vi "Write Valve Parameters.vi"(7 "listen period":sgl=0.1, 8 "error in":errorcluster, 9 "Valve Range":i32=5391, 10 "Valve Offset":i32=13225, 11 "Brooks MFC in":refnum<class "Brooks MFC.lvclass">) -> (0 "error out":errorcluster, 1 "Valve Range":i32=5391, 2 "Valve Offset":i32=13225, 3 "Brooks MFC out":refnum<class "Brooks MFC.lvclass">)   [LabVIEW 2016, in "Brooks MFC.lvclass"]
uses:
  Brooks MFC.lvclass
  Brooks MFC.lvclass/Brooks MFC.ctl
  Instance           5 30Saved   Write Valve Parameters .vi
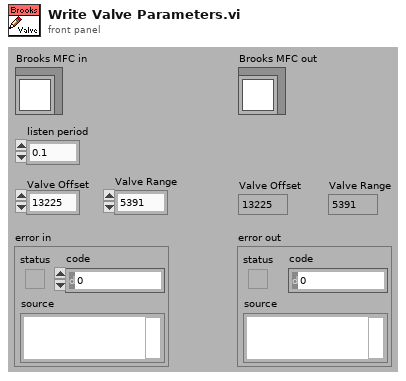
[diagram p1: front panel]
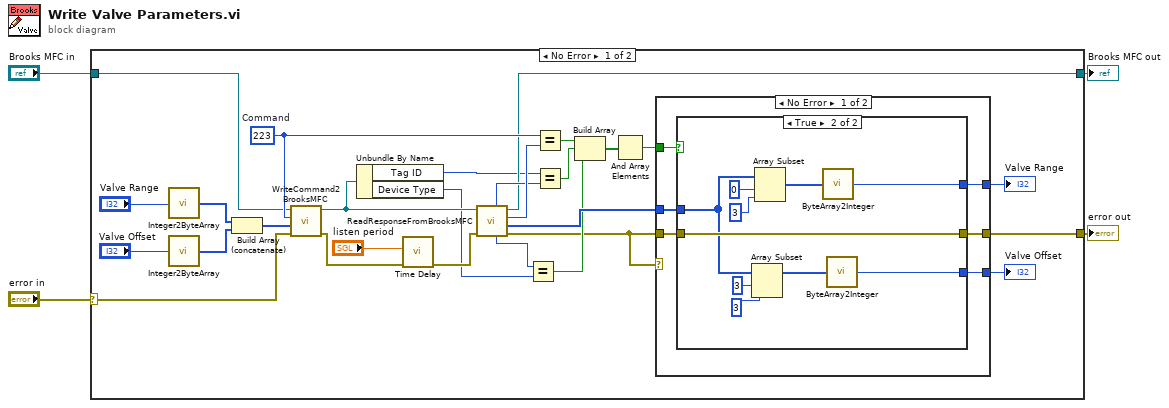
[diagram p0: block diagram]
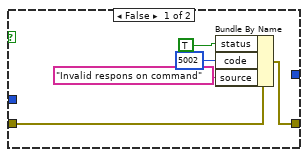
[diagram p2: hidden frame]
diagram:
  n1 = case shown="No Error" "error in" {
    selector: "error in" -> [w10 w55]
    tunnel: "Brooks MFC in" -> [w11 w56]
    tunnel: [w8 w56] -> w2
    tunnel: [w9 w55] -> w1
    frame No Error {
      w14 = u8 223  # Command
      n2 = call "Integer2ByteArray.vi"("Integer"="Valve Range") -> ("Byte Array"=w30:u8[])
      n3 = call "Integer2ByteArray.vi"("Integer"="Valve Offset") -> ("Byte Array"=w29:u8[])
      n4 = Build Array (concatenate)(w30, w29) -> (w13:u8[])
      n5 = call "WriteCommand2BrooksMFC.vi"("error in"=w10, "Data"=w13, "Command"=w14, "Brooks MFC in"=w11) -> ("error out"=w24:errorcluster, "Brooks MFC out"=w7:refnum<class "Brooks MFC.lvclass">)  [unwired: 5 in, 1 out]
      n6 = Unbundle By Name(w7) -> ("Tag ID"=w6:u32, "Device Type"=w5:u8)
      n7 = call "Time Delay"("error in (no error)"=w24, "Delay Time (s)"="listen period") -> ("error out"=w23:errorcluster)  [unwired: 9 in]
      n8 = call "ReadResponseFromBrooksMFC.vi"("error in"=w23, "Brooks MFC in"=w7) -> ("error out"=w12:errorcluster, "Data"=w28:u8[], "Command"=w25:u8, "Brooks MFC out"=w8:refnum<class "Brooks MFC.lvclass">, "device type"=w20:u8, "tag ID"=w21:u32)  [unwired: 4 in]
      n9 = Equal?(x=w20, y=w5) -> (x = y?=w15:bool)
      n10 = Equal?(x=w14, y=w25) -> (x = y?=w19:bool)
      n11 = Equal?(x=w6, y=w21) -> (x = y?=w16:bool)
      n12 = Build Array(w19, w16, w15) -> (w18:bool[])
      n13 = And Array Elements(Boolean array=w18) -> (logical AND=w17:bool)
      n14 = case shown="No Error" w12 {
        tunnel: w12 -> [w38 w54]
        tunnel: w28 -> [w37 _]
        tunnel: [w36 w54] -> w9
        tunnel: [w35 _] -> w27
        tunnel: [w34 _] -> w26
        tunnel: w17 -> [w33 _]
        frame No Error {
          n15 = case shown="True" w33 {
            tunnel: w37 -> [_ w50]
            tunnel: w38 -> [w40 w51]
            tunnel: [w39 w51] -> w36
            tunnel: [_ w45] -> w35
            tunnel: [_ w46] -> w34
            frame False {
              n16 = Bundle By Name(cluster=w40, "status"=TRUE ("Bundle Element"), "code"=5002 ("Bundle Element"), "source"="Invalid respons on command" ("Bundle Element")) -> (w39:errorcluster)
            }
            frame True {
              n17 = Array Subset(array=w50, index=3 ("Array Index"), length=3 ("Array Length")) -> (w44:u8[])
              n18 = Array Subset(array=w50, index=0 ("Index"), length=3) -> (w47:u8[])
              n19 = call "ByteArray2Integer.vi"("Byte Array"=w47) -> ("Integer"=w46:u32)
              n20 = call "ByteArray2Integer.vi"("Byte Array"=w44) -> ("Integer"=w45:u32)
            }
          }
        }
        frame Error {
        }
      }
      "Valve Range" <- w26
      "Valve Offset" <- w27
    }
    frame Error {
    }
  }
  "Brooks MFC out" <- w2
  "error out" <- w1
